vi "MotionProfileGenerator.vi"(1 "MotionProfileGeneratorParameters":T1={"Trajectory Point Interval (ms)"=10, "Maximum Travel Speed (units/s)"=0.0, "Velocity Ramp Time (ms)"=0.0, "Acceleration Ramp Time (ms)"=1.0} {"Acceleration Ramp Time (ms)" min=1.0; "Velocity Ramp Time (ms)" min=1.0; "Maximum Travel Speed (units/s)" min=0.0; "Trajectory Point Interval (ms)" items=["TrajectoryDuration_0ms"=0, "TrajectoryDuration_5ms"=5, "TrajectoryDuration_10ms"=10, "TrajectoryDuration_20ms"=20, "TrajectoryDuration_30ms"=30, "TrajectoryDuration_40ms"=40, "TrajectoryDuration_50ms"=50, "TrajectoryDuration_100ms"=100]}, 2 "Starting Position (units)":dbl, 3 "Travel Distance (units)":dbl) -> (0 "Trajectory Points":T3[](array[typedef]) {"Time (ms)" items=["TrajectoryDuration_0ms"=0, "TrajectoryDuration_5ms"=5, "TrajectoryDuration_10ms"=10, "TrajectoryDuration_20ms"=20, "TrajectoryDuration_30ms"=30, "TrajectoryDuration_40ms"=40, "TrajectoryDuration_50ms"=50, "TrajectoryDuration_100ms"=100]})   [LabVIEW 2018]
uses:
  TypeDefs/TrajectoryPoint.ctl
  <vilib>/Rock Robotics/WPI/ThirdParty/Phoenix-LabVIEW/Motor Controller/Controls/CTRE_Phoenix_MotorControl_TrajectoryPointTimeDur.ctl
  TypeDefs/MotionProfileGeneratorParams.ctl
  ArgosLib/ArgosLib.lvlib
panel:
  out "Input":bool
  out "T4":dbl
  out "fl2":dbl
  out "fl1":dbl
  out "n":dbl
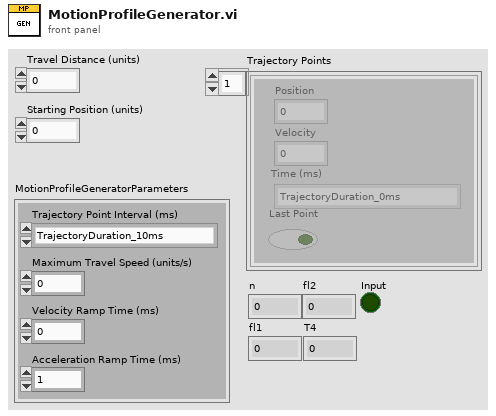
[diagram p1: front panel]
types:
  T1 = typedef "MotionProfileGeneratorParams.ctl" = cluster{"Trajectory Point Interval (ms)":T2, "Maximum Travel Speed (units/s)":dbl, "Velocity Ramp Time (ms)":dbl, "Acceleration Ramp Time (ms)":dbl}
  T2 = typedef "CTRE_Phoenix_MotorControl_TrajectoryPointTimeDur.ctl" = i32
  T3 = typedef "TrajectoryPoint.ctl" = cluster{"Position ":dbl, "Velocity ":dbl, "Time (ms)":T2, "Last Point":bool}
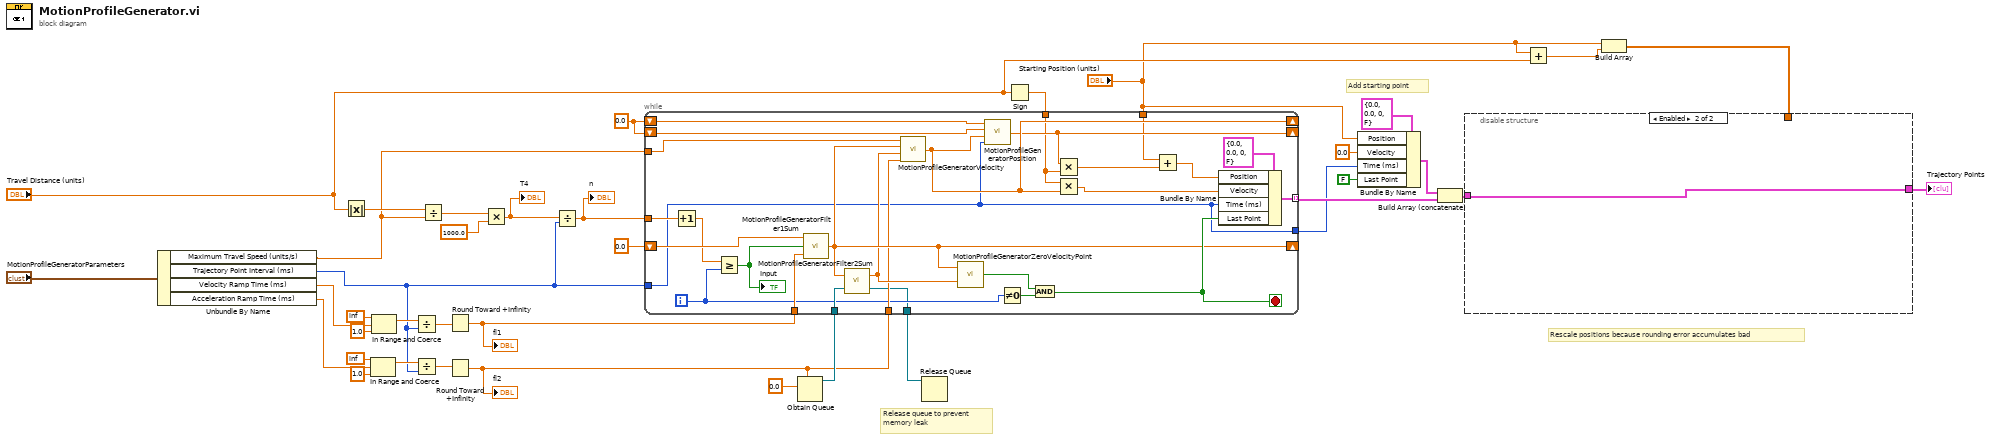
[diagram p0: block diagram]
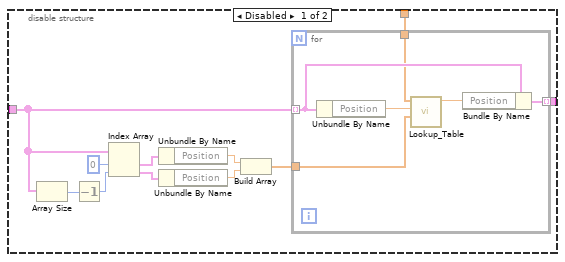
[diagram p2: hidden frame]
diagram:
  w20 = 0.0
  # "Rescale positions because rounding error accumulates bad"
  # "Release queue to prevent\nmemory leak"
  # "Add starting point"
  n1 = Unbundle By Name("MotionProfileGeneratorParameters") -> ("Maximum Travel Speed (units/s)"=w7:dbl, "Trajectory Point Interval (ms)"=w17:T2, "Velocity Ramp Time (ms)"=w16:dbl, "Acceleration Ramp Time (ms)"=w15:dbl)
  n2 = Absolute Value(x="Travel Distance (units)") -> (abs(x)=w29:dbl)
  n3 = In Range and Coerce(upper limit=inf, x=w15, lower limit=1.0) -> (coerced(x)=w25:dbl)  [unwired: 1 out]
  n4 = In Range and Coerce(upper limit=inf, x=w16, lower limit=1.0) -> (coerced(x)=w26:dbl)  [unwired: 1 out]
  n5 = Divide(x=w26, y=w17) -> (x/y=w35:dbl)
  n6 = Divide(x=w25, y=w17) -> (x/y=w36:dbl)
  n7 = Divide(x=w29, y=w7) -> (x/y=w38:dbl)
  n8 = Round Toward +Infinity(x=w35) -> (ceil(x): smallest int >= x=w28:dbl)
  "fl1" <- w28
  n9 = Round Toward +Infinity(x=w36) -> (ceil(x): smallest int >= x=w27:dbl)
  "fl2" <- w27
  n10 = Multiply(x=w38, y=1000.0) -> (x*y=w34:dbl)
  "T4" <- w34
  n11 = Divide(x=w34, y=w17) -> (x/y=w33:dbl)
  "n" <- w33
  n12 = Obtain Queue(max queue size (-1, unlimited)=w27, element data type=0.0) -> (queue out=w30:refnum<queue>)  [unwired: 3 in, 2 out]
  n13 = Sign(1:"Travel Distance (units)") -> (0:w19:dbl)
  n14 = while {
    tunnel: w17 -> [w39]
    tunnel: w33 -> [w65]
    shift-right: [w54] -> _
    shift-left: 0.0 -> [w56]
    tunnel: w30 -> [w58]
    tunnel: [w62] -> w9 mode=indexing
    tunnel: w27 -> [w52]
    tunnel: w7 -> [w55]
    shift-right: [w47] -> _
    shift-left: w20 -> [w60]
    shift-right: [w45] -> _
    shift-left: w20 -> [w51]
    tunnel: w28 -> [w57]
    tunnel: w19 -> [w44]
    tunnel: [w41] -> w14
    tunnel: "Starting Position (units)" -> [w40]
    tunnel: [w39] -> w8
    i -> [w50]
    stop <- w61 stop-if-true
    n15 = Increment(x=w65) -> (x+1=w49:dbl)
    n16 = Greater Or Equal?(x=w49, y=w50) -> (x >= y?=w48:bool)
    "Input" <- w48
    n17 = call "MotionProfileGeneratorFilter1Sum.vi"("fl1"=w57, "Input"=w48, "Previous Filter1Sum"=w56) -> ("Filter1Sum"=w54:dbl)
    n18 = call "MotionProfileGeneratorFilter2Sum.vi"("Filter Queue"=w58, "Filter1Sum"=w54) -> ("queue out"=w41:refnum<queue>, "Filter2Sum"=w53:dbl)
    n19 = call "MotionProfileGeneratorVelocity.vi"("FL2"=w52, "filter2sum"=w53, "Filter1Sum"=w54, "Maximum Travel Speed (rps)"=w55) -> ("Velocity"=w47:dbl)
    n20 = call "MotionProfileGeneratorZeroVelocityPoint.vi"("Filter2Sum"=w53, "Filter1Sum"=w54) -> ("Zero Velocity"=w59:bool)
    n21 = call "MotionProfileGeneratorPosition.vi"("Trajectory Point Interval (ms)"=w39, "Velocity"=w47, "Previous Position"=w51, "Previous Velocity"=w60) -> ("Position"=w45:dbl)
    n22 = Not Equal To 0?(x=w50) -> (x != 0?=w64:bool)
    n23 = And(x=w59, y=w64) -> (x .and. y?=w61:bool)
    n24 = Multiply(x=w45, y=w44) -> (x*y=w43:dbl)
    n25 = Multiply(x=w44, y=w47) -> (x*y=w46:dbl)
    n26 = Add(x=w40, y=w43) -> (x+y=w42:dbl)
    n27 = Bundle By Name(cluster=T3 {"Position "=0.0, "Velocity "=0.0, "Time (ms)"=0, "Last Point"=FALSE} ("trajectory point"), "Position"=w42, "Velocity"=w46, "Time (ms)"=w39, "Last Point"=w61) -> (w62:T3)
  }
  n28 = Release Queue(queue=w14) -> ()  [unwired: 2 in, 3 out]
  n29 = Bundle By Name(cluster=T3 {"Position "=0.0, "Velocity "=0.0, "Time (ms)"=0, "Last Point"=FALSE} ("trajectory point"), "Position"="Starting Position (units)", "Velocity"=0.0, "Time (ms)"=w8, "Last Point"=FALSE) -> (w12:T3)
  n30 = Build Array (concatenate)(w12, w9) -> (w1:T3[])
  n31 = Add(x="Starting Position (units)", y="Travel Distance (units)") -> (x+y=w3:dbl)
  n32 = Build Array("Starting Position (units)", w3) -> (w2:dbl[])
  n33 = disable-structure shown="Enabled" {
    disable-tunnel: [w76 w83] -> w6
    disable-tunnel: w2 -> [w67 _]
    disable-tunnel: w1 -> [w75 w83]
    frame Disabled {
      n34 = Array Size(array=w75) -> (size(s)=w74:i32)
      n35 = Decrement(x=w74) -> (x-1=w73:i32)
      n36 = Index Array(array=w75, index #1=0 ("index"), index #2=w73) -> (element #1=w71:T3, element #2=w70:T3)
      n37 = Unbundle By Name(w71) -> ("Position"=w69:dbl)
      n38 = Unbundle By Name(w70) -> ("Position"=w68:dbl)
      n39 = Build Array(w69, w68) -> (w66:dbl[])
      n40 = for {
        tunnel: w75 -> [w81] mode=indexing
        tunnel: [w79] -> w76 mode=indexing
        tunnel: w67 -> [w78]
        tunnel: w66 -> [w77]
        n41 = Unbundle By Name(w81) -> ("Position"=w82:dbl)
        n42 = call "Lookup_Table.vi"("Y_Array"=w78, "x_in"=w82, "X_Array"=w77) -> ("y_out"=w80:dbl)  [unwired: 6 in]
        n43 = Bundle By Name(cluster=w81, "Position"=w80) -> (w79:T3)
      }
    }
    frame Enabled {
    }
  }
  "Trajectory Points" <- w6
